vi "ModifyChnlHW.vi"(8 "error in (no error)":errorcluster, 11 "BME_DG_G02_Chnl in":refnum<class "BME_DG_G02_Chnl.lvclass">) -> (0 "error out":errorcluster, 3 "BME_DG_G02_Chnl out":refnum<class "BME_DG_G02_Chnl.lvclass">)   [LabVIEW 2009, in "BME_DG_G02_Chnl.lvclass"]
uses:
  BME_DG_G02_Chnl.lvclass
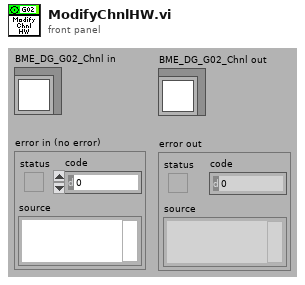
[diagram p1: front panel]
types:
  T1 = typedef "ChnlSettings.ctl" = cluster{" Delay (µs)":dbl, "On? (false)":bool, "PositiveVoltage?(true)":bool, "50OhmTerminated? ":bool, "25OhmOutput?":bool}
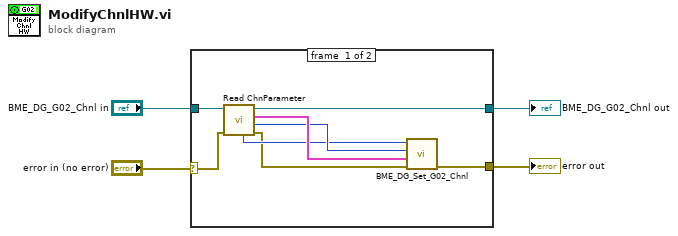
[diagram p0: block diagram]
diagram:
  n1 = case shown="No Error" "error in (no error)" {
    selector: "error in (no error)" -> [w7 w14]
    tunnel: [w5 w14] -> w1
    tunnel: [w10 w13] -> w3
    tunnel: "BME_DG_G02_Chnl in" -> [w11 w13]
    frame #0 {
      n2 = call-dynamic "Read ChnParameter.vi"("error in (no error)"=w7, "BME_DG_Chnl in"=w11) -> ("error out"=w6:errorcluster, "Nr"=w9:i32, "ChnParemater"=w12:T1, "BME_DG_Chnl out"=w10:refnum<class "BME_DG_G02_Chnl.lvclass">, "DG Nr"=w8:i32)  [unwired: 4 in, 1 out]
      n3 = call "BME_DG_Set_G02_Chnl.vi"("error in (no error)"=w6, "ChnParemater"=w12, "Channel"=w9, "DG_Number"=w8) -> ("error out"=w5:errorcluster)  [unwired: 6 in, 1 out]
    }
    frame #1 {
    }
  }
  "error out" <- w1
  "BME_DG_G02_Chnl out" <- w3
